vi "MonitorCurrent.vi"() -> ()   [LabVIEW 2014]
uses:
  <userlib>/Nanonis Prog Interface V5/Nanonis Prog Interface.lvlib
panel:
  in  "trigger interval":u32=5
  out "Current #2":sgl=-2.500167e-11 format="%#_6p"
  out "Current #1":sgl=-2.4994994e-11 format="%#_6p"
  in  "sent interval [s]":u32=600
  in  "threshold":sgl=3e-09 format="%#_6p"
  in  "stop":bool
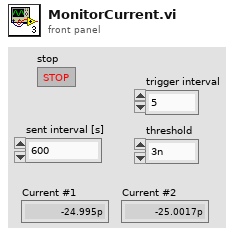
[diagram p1: front panel]
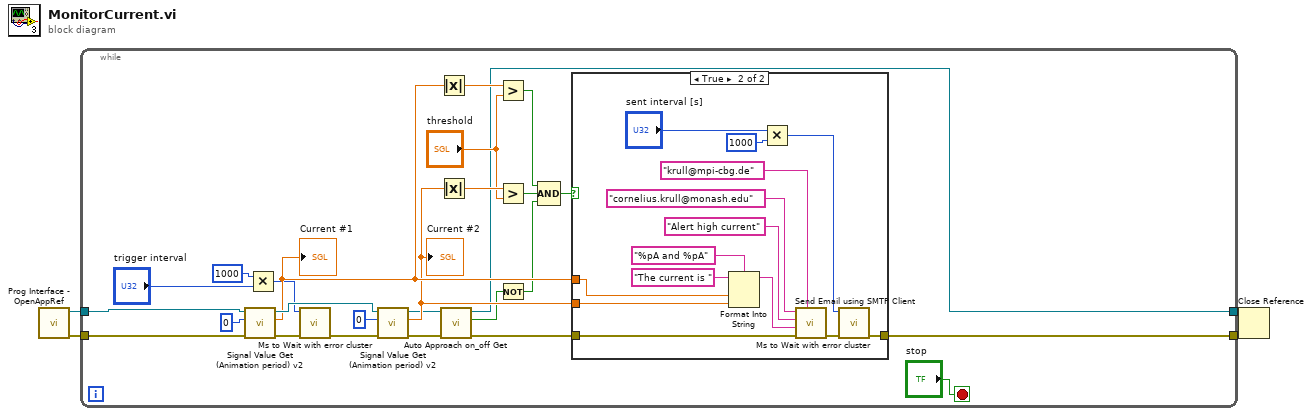
[diagram p0: block diagram]
diagram:
  n1 = call <userlib>:"Prog Interface - OpenAppRef.vi"() -> ("Error out"=w3:errorcluster, "Application reference"=w4:refnum<vi>)  [unwired: 6 in]
  n2 = while {
    tunnel: [w13] -> w1
    tunnel: w4 -> [w12]
    tunnel: w3 -> [w11]
    tunnel: [w9] -> w2
    stop <- "stop" stop-if-true
    n3 = call <userlib>:"Signal Value Get (Animation period) v2.vi"("error in (no error)"=w11, "Signal index (0-79)"=i8 0, "Application ref in"=w12) -> ("error out"=w27:errorcluster, "Signal value"=w18:sgl, "Application ref out"=w25:refnum<vi>)  [unwired: 5 in]
    "Current #1" <- w18
    n4 = Multiply(x=u32 1000, y="trigger interval") -> (x*y=w15:u32)
    n5 = call <userlib>:"Ms to Wait with error cluster.vi"("error in (no error)"=w27, "milliseconds to wait"=w15) -> ("error out"=w26:errorcluster)  [unwired: 4 in, 1 out]
    n6 = call <userlib>:"Signal Value Get (Animation period) v2.vi"("error in (no error)"=w26, "Signal index (0-79)"=i8 0, "Application ref in"=w25) -> ("error out"=w6:errorcluster, "Signal value"=w17:sgl, "Application ref out"=w10:refnum<vi>)  [unwired: 5 in]
    "Current #2" <- w17
    n7 = Absolute Value(x=w18) -> (abs(x)=w28:sgl)
    n8 = Absolute Value(x=w17) -> (abs(x)=w23:sgl)
    n9 = call <userlib>:"Auto Approach on_off Get.vi"("Error in (no error)"=w6, "Application ref in"=w10) -> ("Error out"=w5:errorcluster, "Auto approach on/off status"=w8:bool, "Application ref out"=w9:refnum<vi>)  [unwired: 5 in]
    n10 = Greater?(x=w28, y="threshold") -> (0:w21:bool)
    n11 = Greater?(x=w23, y="threshold") -> (0:w20:bool)
    n12 = Not(x=w8) -> (.not. x?=w7:bool)
    n13 = Compound Arithmetic op=AND(w21, w20, w7) -> (w19:bool)
    n14 = case shown="True" w19 {
      tunnel: w18 -> [_ w40]
      tunnel: w17 -> [_ w39]
      tunnel: w5 -> [w31 w38]
      tunnel: [w31 w36] -> w13
      frame False {
      }
      frame True {
        n15 = Format Into String(format string="%pA and %pA", initial string="The current is ", w40, w39) -> (resulting string=w41:string)  [unwired: 1 in, 1 out]
        n16 = Multiply(x="sent interval [s]", y=u32 1000 ("milliseconds to wait")) -> (x*y=w33:u32)
        n17 = call "Send Email using SMTP Client.vi"("CC"="krull@mpi-cbg.de" ("To:"), "error in (no error)"=w38, "Message"=w41, "Subject"="Alert high current", "To:"="cornelius.krull@monash.edu") -> ("error out"=w37:errorcluster)  [unwired: 6 in]
        n18 = call <userlib>:"Ms to Wait with error cluster.vi"("error in (no error)"=w37, "milliseconds to wait"=w33) -> ("error out"=w36:errorcluster)  [unwired: 4 in, 1 out]
      }
    }
  }
  n19 = Close Reference(reference=w2, error in (no error)=w1) -> ()  [unwired: 1 out]
